vi "Initialize.vi"(8 "error in":errorcluster, 11 "Plugin in":refnum<class "DFT_Spectra.lvclass">) -> (0 "error out":errorcluster, 3 "Plugin out":refnum<class "DFT_Spectra.lvclass">)   [LabVIEW 2024, in "DFT_Spectra.lvlib" / "DFT_Spectra.lvclass"]
uses:
  DFT_Spectra.lvclass
  C:/Program Files/National Instruments/LabVIEW 2024/vi.lib/FlexLogger/SDK/PluginSDK.lvlibp/PEFClasses/SDK/Plugin/Plugin.lvclass
  DFT_Spectra Global.vi
  <vilib>/FlexLogger/SDK/PluginSDK.lvlibp/PEFClasses/SDK/Plugin/ParameterAccess/Write N Channel.vi
  <vilib>/FlexLogger/SDK/PluginSDK.lvlibp/PEFClasses/SDK/Plugin/ParameterAccess/Write DBL.vi
  <vilib>/FlexLogger/SDK/PluginSDK.lvlibp/PEFClasses/SDK/Plugin/ParameterAccess/Write Enum.vi
  <vilib>/FlexLogger/SDK/PluginSDK.lvlibp/PEFClasses/SDK/Plugin/ParameterAccess/Write I32.vi
  <vilib>/FlexLogger/SDK/PluginSDK.lvlibp/PEFClasses/SDK/Plugin/ParameterAccess/Write Command.vi
  <vilib>/FlexLogger/SDK/PluginSDK.lvlibp/PEFClasses/SDK/Plugin/Plugin.lvclass
  C:/Program Files/National Instruments/LabVIEW 2024/vi.lib/FlexLogger/SDK/PluginSDK.lvlibp/PEFClasses/SDK/Processing Element/Processing Element.lvclass
  C:/dev/niflexlogger-plugins/PDK plugins/DFT_Spectra/source/DFT_Spectra.lvclass
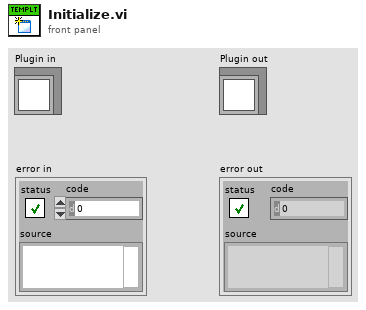
[diagram p1: front panel]
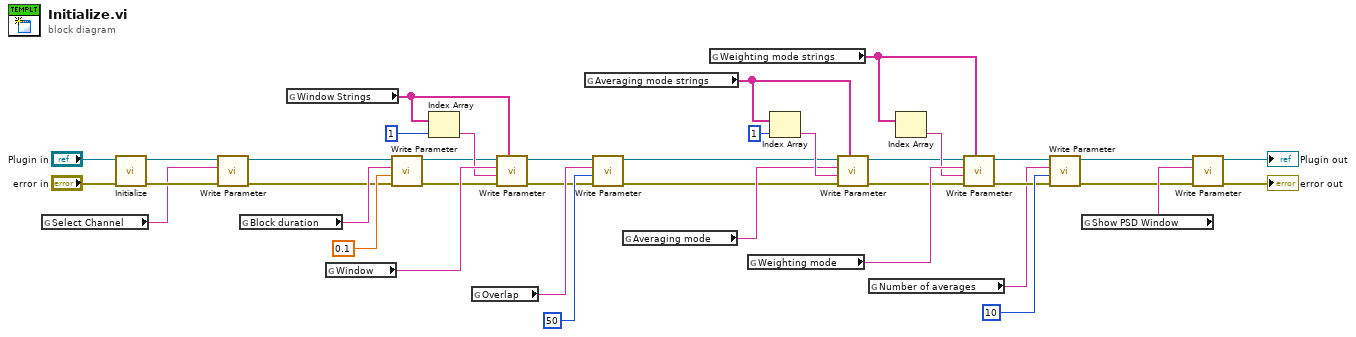
[diagram p0: block diagram]
diagram:
  n1 = global read "DFT_Spectra Global.vi" "Select Channel"() -> (w34:string)
  n2 = call-parent "Initialize.vi"("error in (no error)"="error in", "Plugin in"="Plugin in") -> ("error out"=w35:errorcluster, "Plugin out"=w36:refnum<class "DFT_Spectra.lvclass">)  [unwired: 8 in]
  n3 = call-poly <vilib>:"Write Parameter.vi"("error in (no error)"=w35, "Name (Unique Channel Identifier)"=w34, "Plugin in"=w36) -> ("error out"=w10:errorcluster, "Plugin out"=w11:refnum<class "DFT_Spectra.lvclass">)  [unwired: 7 in]
  n4 = global read "DFT_Spectra Global.vi" "Block duration"() -> (w14:string)
  n5 = global read "DFT_Spectra Global.vi" "Window Strings"() -> (w30:string[])
  n6 = global read "DFT_Spectra Global.vi" "Window"() -> (w31:string)
  n7 = call-poly <vilib>:"Write Parameter.vi"("error in (no error)"=w10, "Value"=0.1, "Name"=w14, "Plugin in"=w11) -> ("error out"=w8:errorcluster, "Plugin out"=w9:refnum<class "DFT_Spectra.lvclass">)  [unwired: 6 in]
  n8 = Index Array(array=w30, index=1) -> (element=w29:string)
  n9 = global read "DFT_Spectra Global.vi" "Overlap"() -> (w17:string)
  n10 = call-poly <vilib>:"Write Parameter.vi"("Possible Values"=w30, "error in (no error)"=w8, "Current Value"=w29, "Name"=w31, "Plugin in"=w9) -> ("error out"=w6:errorcluster, "Plugin out"=w7:refnum<class "DFT_Spectra.lvclass">)  [unwired: 5 in]
  n11 = global read "DFT_Spectra Global.vi" "Averaging mode strings"() -> (w27:string[])
  n12 = call-poly <vilib>:"Write Parameter.vi"("error in (no error)"=w6, "Value"=50, "Name"=w17, "Plugin in"=w7) -> ("error out"=w4:errorcluster, "Plugin out"=w5:refnum<class "DFT_Spectra.lvclass">)  [unwired: 6 in]
  n13 = global read "DFT_Spectra Global.vi" "Averaging mode"() -> (w26:string)
  n14 = global read "DFT_Spectra Global.vi" "Weighting mode strings"() -> (w24:string[])
  n15 = global read "DFT_Spectra Global.vi" "Weighting mode"() -> (w25:string)
  n16 = Index Array(array=w27, index=1) -> (element=w28:string)
  n17 = call-poly <vilib>:"Write Parameter.vi"("Possible Values"=w27, "error in (no error)"=w4, "Current Value"=w28, "Name"=w26, "Plugin in"=w5) -> ("error out"=w21:errorcluster, "Plugin out"=w22:refnum<class "DFT_Spectra.lvclass">)  [unwired: 5 in]
  n18 = global read "DFT_Spectra Global.vi" "Number of averages"() -> (w18:string)
  n19 = Index Array(array=w24) -> (element=w23:string)  [unwired: 1 in]
  n20 = call-poly <vilib>:"Write Parameter.vi"("Possible Values"=w24, "error in (no error)"=w21, "Current Value"=w23, "Name"=w25, "Plugin in"=w22) -> ("error out"=w19:errorcluster, "Plugin out"=w20:refnum<class "DFT_Spectra.lvclass">)  [unwired: 5 in]
  n21 = call-poly <vilib>:"Write Parameter.vi"("error in (no error)"=w19, "Value"=10, "Name"=w18, "Plugin in"=w20) -> ("error out"=w2:errorcluster, "Plugin out"=w3:refnum<class "DFT_Spectra.lvclass">)  [unwired: 6 in]
  n22 = global read "DFT_Spectra Global.vi" "Show PSD Window"() -> (w15:string)
  n23 = call-poly <vilib>:"Write Parameter.vi"("error in (no error)"=w2, "Name"=w15, "Plugin in"=w3) -> ("error out"=→"error out":errorcluster, "Plugin out"=→"Plugin out":refnum<class "DFT_Spectra.lvclass">)  [unwired: 7 in]
